vi "moving_average.vi"(9 "window size":i32=5, 11 "X":dbl[](array[numeric])) -> (3 "averaged X":dbl[](array[numeric]))   [LabVIEW 2020]
uses:
  <vilib>/Analysis/3filter.llb/FIR Filter (DBL).vi
  <vilib>/Analysis/NI_AALBase.lvlib
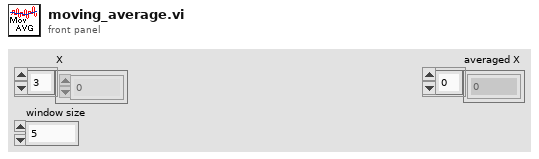
[diagram p1: front panel]
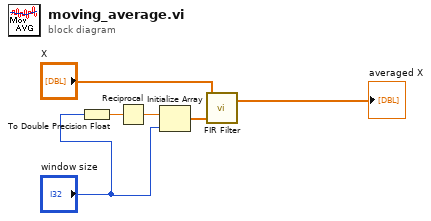
[diagram p0: block diagram]
diagram:
  n1 = To Double Precision Float(number="window size") -> (double precision float=w2:dbl)
  n2 = Reciprocal(x=w2) -> (1/x=w3:dbl)
  n3 = Initialize Array(w3, "window size") -> (w6:dbl[])
  n4 = call-poly <vilib>:"FIR Filter.vi"("FIR Coefficients"=w6, "X"="X") -> ("Filtered X"=→"averaged X":dbl[])  [unwired: 2 in, 1 out]
